vi "Read Volatus INI.vi"(8 "error in (no error)":errorcluster, 10 "INI Path (Default)":path, 11 "Volatus Core in":refnum<class "Volatus Core.lvclass">) -> (0 "error out":errorcluster, 3 "Volatus Core out":refnum<class "Volatus Core.lvclass">)   [LabVIEW 2020, in "Volatus.lvlib" / "Volatus Core.lvclass"]
uses:
  Volatus Core.lvclass
  Volatus Core.lvclass/Volatus Core.ctl
  Volatus.lvlib
  <vilib>/Utility/config.llb/NI_LVConfig.lvlib
  <vilib>/Utility/config.llb/Read Key (String).vi
  Config Type.ctl
  lv-vecto/Vecto/Node Config/Node Info.ctl
  lv-vecto/VectoConfig/VectoConfig.lvlib
  lv-vecto/Vecto/Node Config/Node Config.lvclass
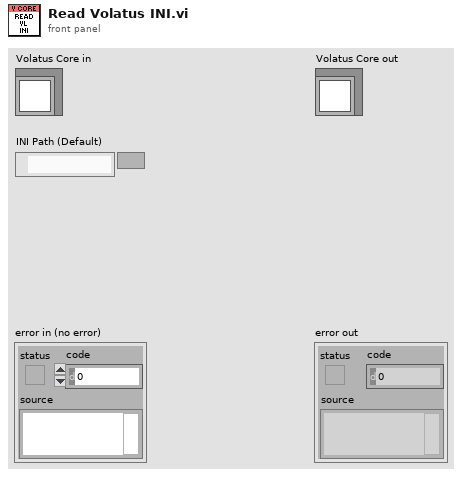
[diagram p1: front panel]
types:
  T1 = typedef "Volatus.lvlib/Volatus Core.lvclass/Config Type.ctl" = enum16{"App INI", "Memory"}
  T2 = typedef "VectoConfig.lvlib/Node Info.ctl" = cluster{"System":string, "Cluster":string, "Name":string, "ID":u32, "Capabilities":string[]}
  T3 = typedef "NI_LVConfig.lvlib/Config Data RefNum.ctl" = refnum<k1>
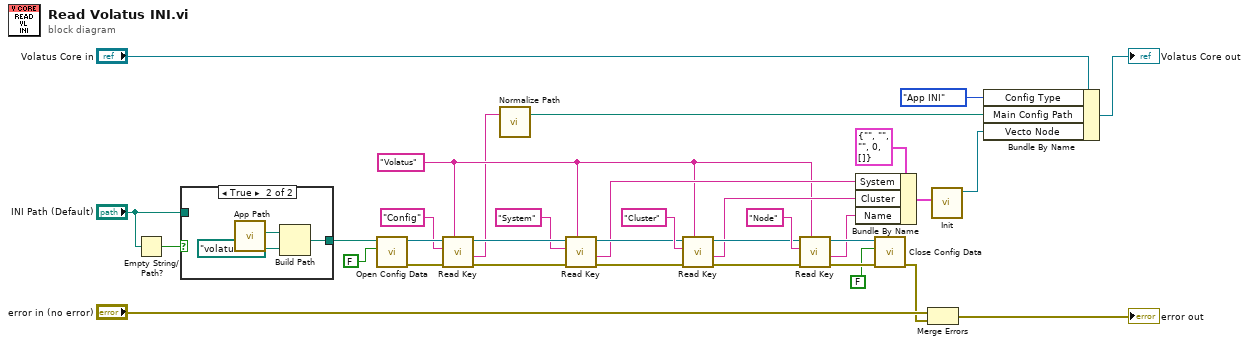
[diagram p0: block diagram]
diagram:
  w6 = "Volatus" ("section")
  n1 = Empty String/Path?(string/path="INI Path (Default)") -> (empty?=w5:bool)
  n2 = case shown="True" w5 {
    tunnel: [w35 w36] -> w33
    tunnel: "INI Path (Default)" -> [w35 _]
    frame False {
    }
    frame True {
      n3 = call "App Path.vi"() -> ("App Path"=w38:path)  [unwired: 11 in]
      n4 = Build Path(base path=w38, name or relative path=path "volatus.ini") -> (appended path=w36:path)
    }
  }
  n5 = call <vilib>:"Open Config Data.vi"("create file if necessary (T)"=FALSE, "configuration file path"=w33) -> ("error out"=w31:errorcluster, "refnum"=w30:T3)  [unwired: 7 in, 1 out]
  n6 = call-poly <vilib>:"Read Key.vi"("section"=w6, "error in (no error)"=w31, "key"="Config" ("section"), "refnum"=w30) -> ("error out"=w26:errorcluster, "value"=w3:string, "refnum out"=w27:T3)  [unwired: 4 in, 1 out]
  n7 = call "Normalize Path.vi"("Path String"=w3) -> ("Path"=w2:path)  [unwired: 2 in]
  n8 = call-poly <vilib>:"Read Key.vi"("section"=w6, "error in (no error)"=w26, "key"="System" ("section"), "refnum"=w27) -> ("error out"=w25:errorcluster, "value"=w14:string, "refnum out"=w24:T3)  [unwired: 4 in, 1 out]
  n9 = call-poly <vilib>:"Read Key.vi"("section"=w6, "error in (no error)"=w25, "key"="Cluster" ("section"), "refnum"=w24) -> ("error out"=w20:errorcluster, "value"=w13:string, "refnum out"=w21:T3)  [unwired: 4 in, 1 out]
  n10 = call-poly <vilib>:"Read Key.vi"("section"=w6, "error in (no error)"=w20, "key"="Node" ("section"), "refnum"=w21) -> ("error out"=w18:errorcluster, "value"=w12:string, "refnum out"=w19:T3)  [unwired: 4 in, 1 out]
  n11 = Bundle By Name(cluster=T2 {"System"="", "Cluster"="", "Name"="", "ID"=0, "Capabilities"=[]} ("Node Info"), "System"=w14, "Cluster"=w13, "Name"=w12) -> (w10:T2)
  n12 = call <vilib>:"Close Config Data.vi"("error in (no error)"=w18, "write file if changed (T)"=FALSE, "refnum"=w19) -> ("error out"=w15:errorcluster)  [unwired: 7 in, 1 out]
  n13 = Merge Errors("error in (no error)", w15) -> (→"error out":errorcluster)
  n14 = call "Init.vi"("Node Info"=w10) -> ("Node out"=w9:refnum<class "Node Config.lvclass">)  [unwired: 9 in, 1 out]
  n15 = Bundle By Name(cluster="Volatus Core in", "Config Type"=Config_Type."App INI", "Main Config Path"=w2, "Vecto Node"=w9) -> (→"Volatus Core out":refnum<class "Volatus Core.lvclass">)
